vi "Arduino - Individual Digital Output Control.vi"() -> ()   [LabVIEW 2011]
doc: "An example that reads a user selectable analog input pin on the Arduino."
uses:
  <vilib>/LabVIEW Interface for Arduino/Type Defs/Connection Type.ctl
  <vilib>/LabVIEW Interface for Arduino/Type Defs/Board Type.ctl
  <vilib>/LabVIEW Interface for Arduino/Type Defs/Pin Mode.ctl
  <vilib>/LabVIEW Interface for Arduino/LabVIEW Interface for Arduino.lvlib
panel:
  out "Port Status Indicator":bool[](array[boolean])
  in  "Arduino Digital Pins (2 to 13)":bool[](array[boolean])
  in  "stop":bool
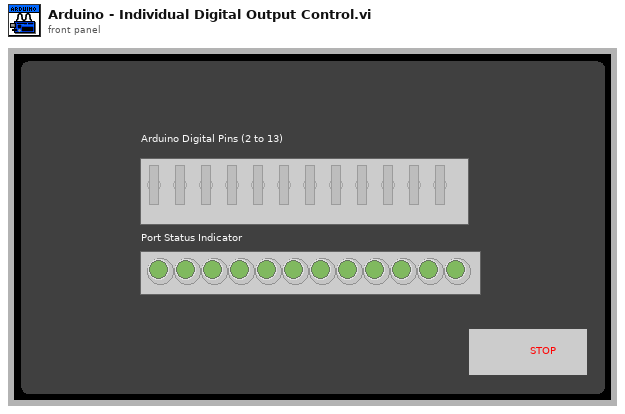
[diagram p1: front panel]
types:
  T1 = typedef "LabVIEW Interface for Arduino.lvlib/Board Type.ctl" = enum16{"Uno", "Mega 2560"}
  T2 = typedef "LabVIEW Interface for Arduino.lvlib/Connection Type.ctl" = enum8{"USB / Serial", "XBEE", "BlueSmirf (Bluetooth)"}
  T3 = typedef "LabVIEW Interface for Arduino.lvlib/Arduino Resource.ctl" = cluster{"VISA resource":refnum<visa-resource-name>, "Board Type":T1, "Connection Type":enum8{"USB / Serial"}, "Bytes Per Packet (15)":u8}
  T4 = typedef "LabVIEW Interface for Arduino.lvlib/Pin Mode.ctl" = enum8{"Input", "Output"}
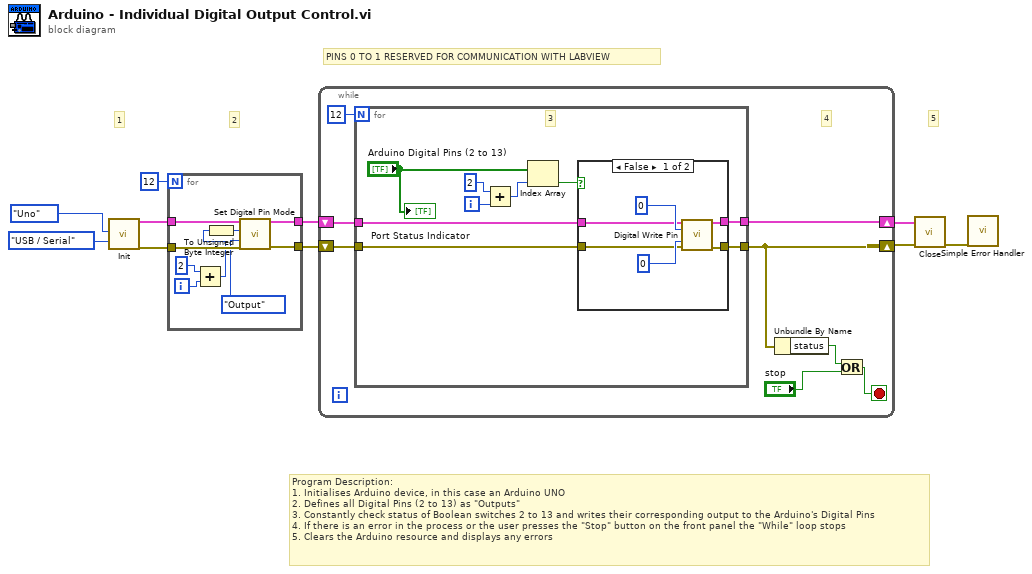
[diagram p0: block diagram]
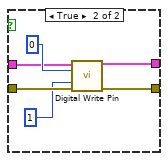
[diagram p2: hidden frame]
diagram:
  # "PINS 0 TO 1 RESERVED FOR COMMUNICATION WITH LABVIEW"
  # "Program Description:\n1. Initialises Arduino device, in this case an Arduino UNO\n2. Defines all Digital Pins (2 to 13) as \"Outputs\"\n3. Constantly check status of Boolean switches 2 to 13 and writes their corresponding output to the Arduino's Digital Pins\n4. If there is an error in the process or the user presses the \"Stop\" button on the front panel the \"While\" loop stops\n5. Clears the Arduino resource and displays any errors"
  # "5"
  # "2"
  # "1"
  n1 = call <vilib>:"Init.vi"("Board Type (Uno)"=Board_Type."Uno", "Connection Type (USB/Serial)"=Connection_Type."USB / Serial") -> ("Arduino Resource"=w5:T3, "error out"=w2:errorcluster)  [unwired: 16 in]
  n2 = for {
    N: 12 -> [_]
    tunnel: w5 -> [w19]
    tunnel: [w18] -> w4
    tunnel: [w17] -> w3
    tunnel: w2 -> [w16]
    i -> [w13]
    n3 = Add(x=2, y=w13) -> (x+y=w11:i32)
    n4 = To Unsigned Byte Integer(number=w11) -> (unsigned 8bit integer=w15:u8)
    n5 = call <vilib>:"Set Digital Pin Mode.vi"("Arduino Resource"=w19, "Digital I/O Pin"=w15, "Pin Mode (Input)"=Pin_Mode."Output", "error in"=w16) -> ("Arduino Resource"=w18:T3, "error out"=w17:errorcluster)  [unwired: 10 in]
  }
  n6 = while {
    shift-right: [w26] -> w10
    shift-left: w4 -> [w21]
    shift-right: [w25] -> w9
    shift-left: w3 -> [w22]
    stop <- w27 stop-if-true
    # "4"
    n7 = for {
      N: 12 -> [_]
      tunnel: [w36] -> w26
      tunnel: [w35] -> w25
      tunnel: w22 -> [w34]
      tunnel: w21 -> [w33]
      i -> [w29]
      # "3"
      n8 = Add(x=2, y=w29) -> (x+y=w28:i32)
      n9 = Index Array(array="Arduino Digital Pins (2 to 13)", index=w28) -> (element=w32:bool)
      n10 = case shown="False" w32 {
        tunnel: w33 -> [w40 w47]
        tunnel: w34 -> [w39 w46]
        tunnel: [w38 w45] -> w36
        tunnel: [w37 w44] -> w35
        frame False {
          n11 = call <vilib>:"Digital Write Pin.vi"("Arduino Resource"=w40, "Digital I/O Pin (0)"=u8 0, "Value (0)"=u8 0, "error in"=w39) -> ("Arduino Resource"=w38:T3, "error out"=w37:errorcluster)  [unwired: 10 in]
        }
        frame True {
          n12 = call <vilib>:"Digital Write Pin.vi"("Arduino Resource"=w47, "Digital I/O Pin (0)"=u8 0, "Value (0)"=u8 1, "error in"=w46) -> ("Arduino Resource"=w45:T3, "error out"=w44:errorcluster)  [unwired: 10 in]
        }
      }
      "Port Status Indicator" <- "Arduino Digital Pins (2 to 13)"
    }
    n13 = Unbundle By Name(w25) -> ("status"=w24:bool)
    n14 = Or(x=w24, y="stop") -> (x .or. y?=w27:bool)
  }
  n15 = call <vilib>:"Close.vi"("Arduino Resource"=w10, "error in"=w9) -> ("error out"=w8:errorcluster)  [unwired: 13 in]
  n16 = call <vilib>:"Simple Error Handler.vi"("error in (no error)"=w8) -> ()  [unwired: 4 in, 5 out]
